vi "GT 2D Compare Pulse.vi"(6 "time":i16, 7 "outputType":i16, 8 "error in (no error)":errorcluster caption="错误输入（无错误）", 9 "level":i16, 10 "chn":i16, 11 "cardNum":i16) -> (0 "error out":errorcluster caption="错误输出", 3 "function return":i16)   [LabVIEW 2014, in "gts.lvlib"]
doc: "GT_API GT_2DComparePulse(short cardNum,short chn,short level,short outputType,short time);"
uses:
  gts.lvlib
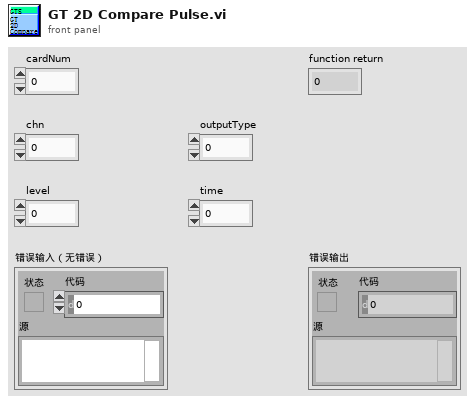
[diagram p1: front panel]
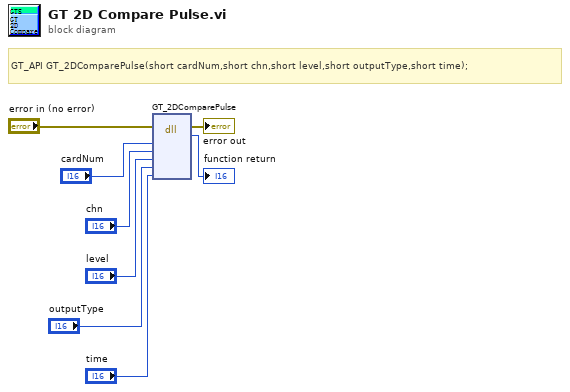
[diagram p0: block diagram]
diagram:
  # "GT_API GT_2DComparePulse(short cardNum,short chn,short level,short outputType,short time);"
  n1 = dll-call lib="PTH2habs D固高科技资料GTS控制卡GTS卡18年上半年资料dllVC32bit\nmulti_cardgts.*" fn="GT_2DComparePulse"(error in="error in (no error)", "cardNum"="cardNum", "chn"="chn", "level"="level", "outputType"="outputType", "time"="time") -> (error out=→"error out":errorcluster, →"function return":i16)  [unwired: 7 in, 1 out]
